vi "2-Position Single Solenoid Control.vi"(6 "Sensor Analog Status":sgl format="%#_13g", 7 "Sensor Digital Status":bool, 9 "Feedback":T5(ring), 10 "Action":T4(ring), 11 "PneumaticsDevRefIn":T1={"Pneumatic State Reference"=refnum, "SolenoidDevRef"={"DevStatus"={"status"=FALSE, "code"=0, "source"=""}, "Pneumatics Control Module"=0, "Forward Solenoid Channel"=enum."Invalid", "Reverse Solenoid Channel"=enum."Invalid"}, "Pneumatic Configuration reference"=refnum}) -> (1 "Action Complete":bool, 2 "Solenoid Position":bool, 3 "PneumaticsDevRefOut":T1={"Pneumatic State Reference"=refnum, "SolenoidDevRef"={"DevStatus"={"status"=FALSE, "code"=0, "source"=""}, "Pneumatics Control Module"=0, "Forward Solenoid Channel"=enum."Invalid", "Reverse Solenoid Channel"=enum."Invalid"}, "Pneumatic Configuration reference"=refnum})   [LabVIEW 2014]
uses:
  <userlib>/836 Library/Pneumatics/Pneumatics/836_PneumaticsDevRef.ctl
  <userlib>/836 Library/Pneumatics/Pneumatics/Pneumatic State.ctl
  <userlib>/836 Library/Pneumatics/Pneumatics/StateMachine.ctl
  <vilib>/Rock Robotics/WPI/Solenoid/WPI_SolenoidDevRef.ctl
  <vilib>/Rock Robotics/WPI/Solenoid/WPI_SolenoidChannel.ctl
  <userlib>/836 Library/Pneumatics/Pneumatics/Pneumatic Configuration.ctl
  <vilib>/Rock Robotics/WPI/Solenoid/WPI_SolenoidValue.ctl
  <vilib>/Rock Robotics/WPI/Solenoid/WPI_SolenoidSetEnum.vi
panel:
  out "error IO":errorcluster
  out "Error Out":errorcluster
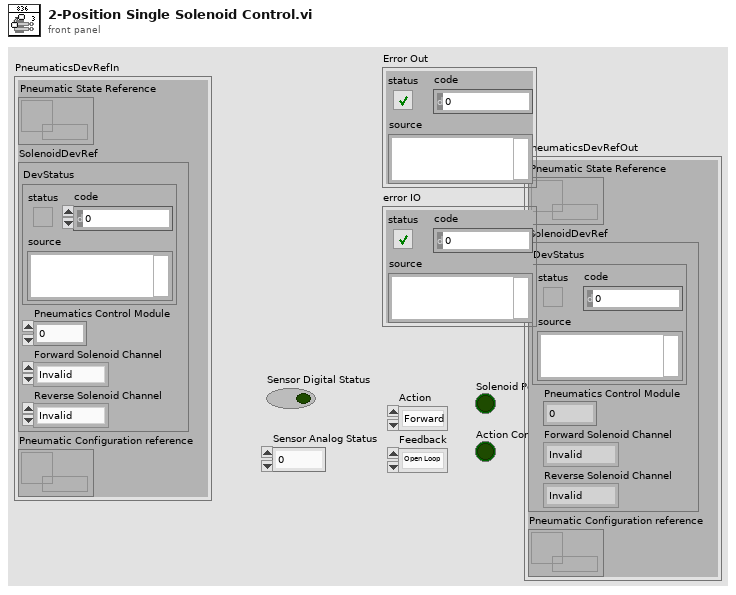
[diagram p1: front panel]
types:
  T1 = typedef "836_PneumaticsDevRef.ctl" = cluster{"Pneumatic State Reference":refnum<data-value>, "SolenoidDevRef":T2, "Pneumatic Configuration reference":refnum<data-value>}
  T2 = typedef "WPI_SolenoidDevRef.ctl" = cluster{"DevStatus":errorcluster, "Pneumatics Control Module":u8, "Forward Solenoid Channel":T3, "Reverse Solenoid Channel":T3}
  T3 = typedef "WPI_SolenoidChannel.ctl" = enum8{"Solenoid 0", "Solenoid 1", "Solenoid 2", "Solenoid 3", "Solenoid 4", "Solenoid 5", "Solenoid 6", "Solenoid 7", "Invalid"}
  T4 = enum16{"Forward", "Back", "Toggle", "Status", "Float"}
  T5 = enum16{"Open Loop", "Analog", "Digital", "Timed"}
  T6 = typedef "WPI_SolenoidValue.ctl" = enum16{"Off", "On", "Forward", "Reverse"}
  T7 = typedef "StateMachine.ctl" = enum8{"Status", "Forward", "Back", "Toggle", "Timed Forward", "Timed Back", "Analog Forwad", "Analog Back", "Digital Forward", "Digital Back", "Off", "Float"}
  T8 = typedef "Pneumatic State.ctl" = cluster{"Position":bool, "Initialize":bool, "Current State":T7, "Multiuse Timer":u32}
  T9 = typedef "Pneumatic Configuration.ctl" = cluster{"Time Forward":u32, "Time Back":u32, "Digital Forward Samples":u32, "Digital Backward Samples":u32, "Analog Forward Settling Time":u32, "Analog Backward Settling Time":u32, "Analog Forward Threshold":sgl, "Analog Backward Threshold":sgl}
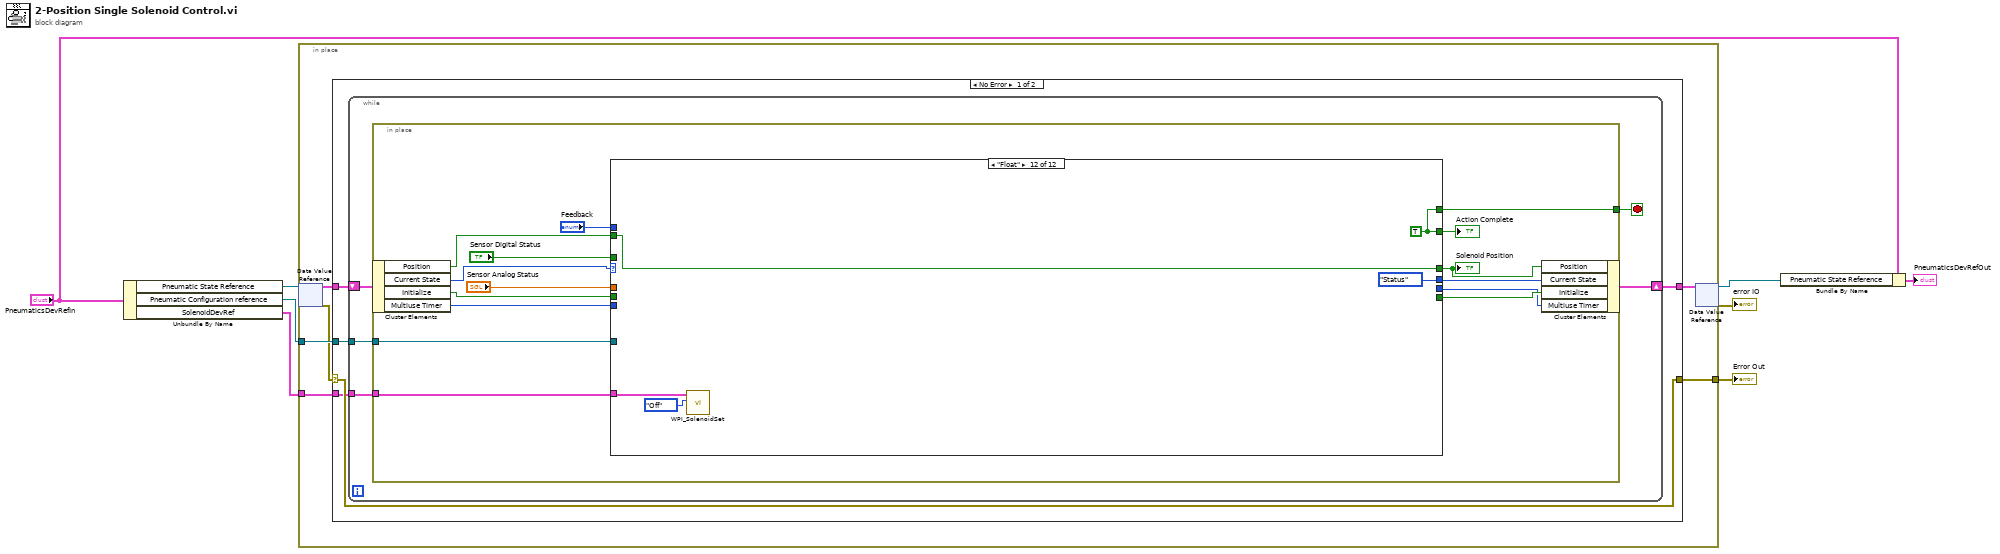
[diagram p0: block diagram]
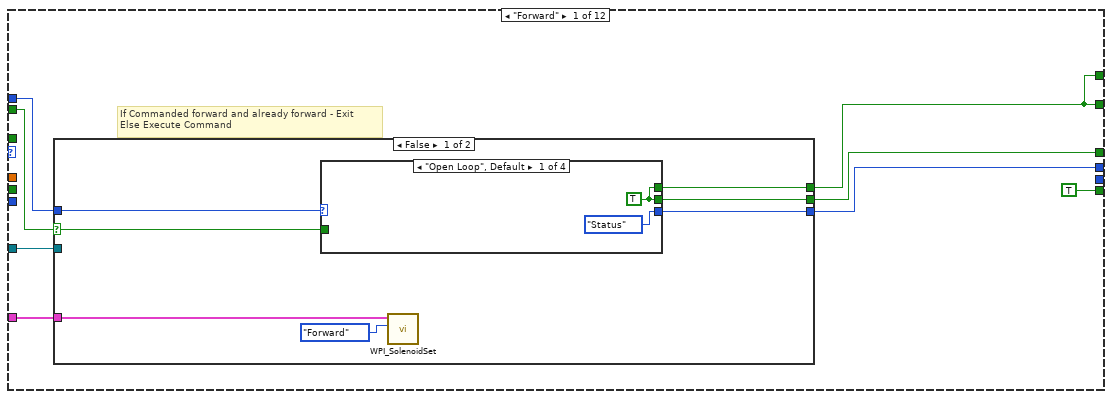
[diagram p2: hidden frame]
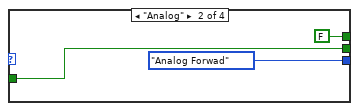
[diagram p3: hidden frame]
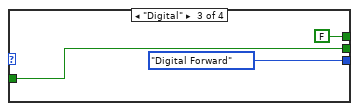
[diagram p4: hidden frame]
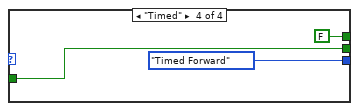
[diagram p5: hidden frame]
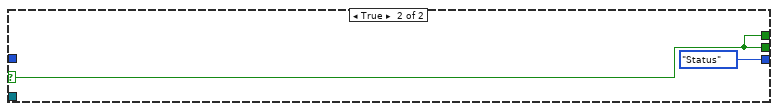
[diagram p6: hidden frame]
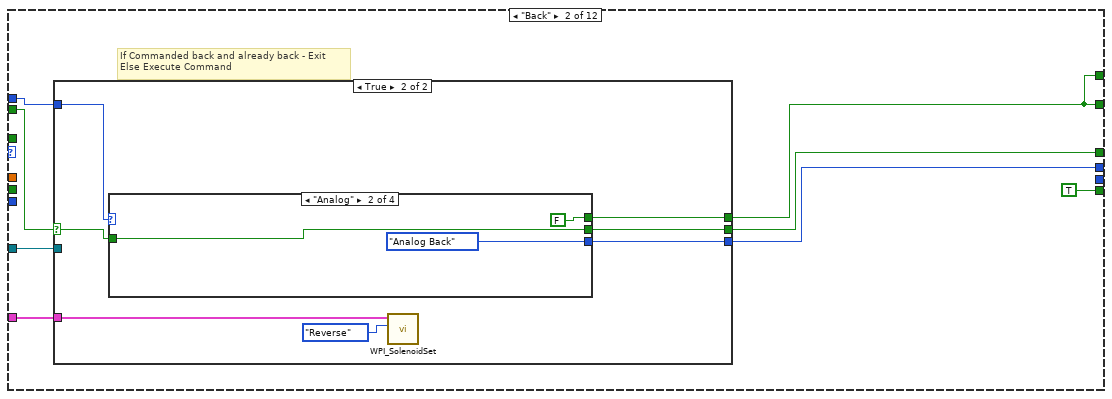
[diagram p7: hidden frame]
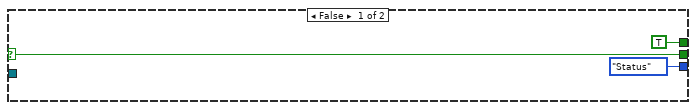
[diagram p8: hidden frame]
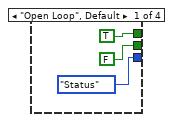
[diagram p9: hidden frame]
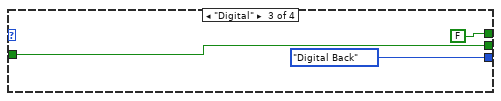
[diagram p10: hidden frame]
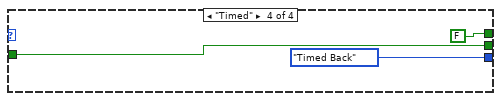
[diagram p11: hidden frame]
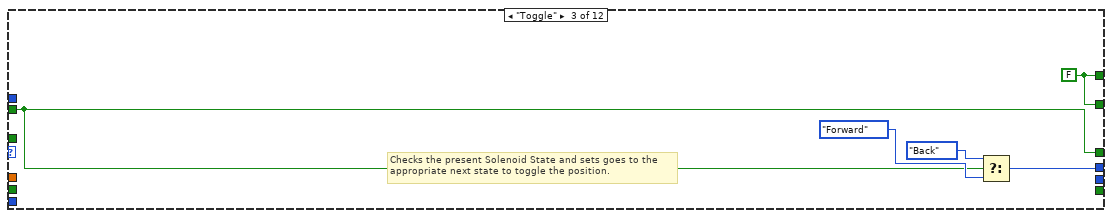
[diagram p12: hidden frame]
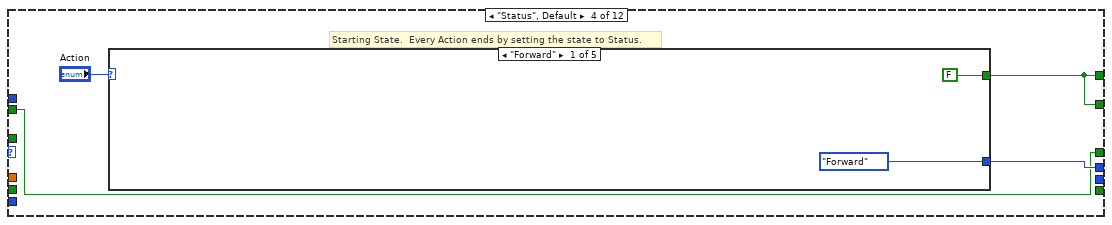
[diagram p13: hidden frame]
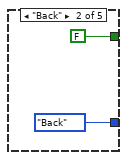
[diagram p14: hidden frame]
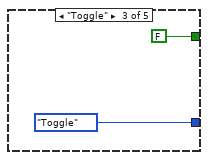
[diagram p15: hidden frame]
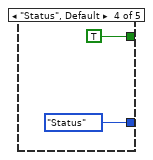
[diagram p16: hidden frame]
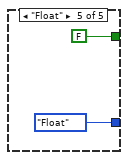
[diagram p17: hidden frame]
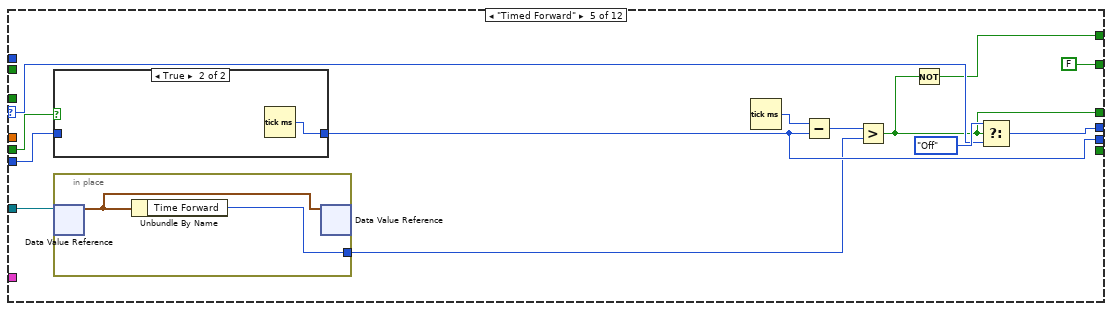
[diagram p18: hidden frame]
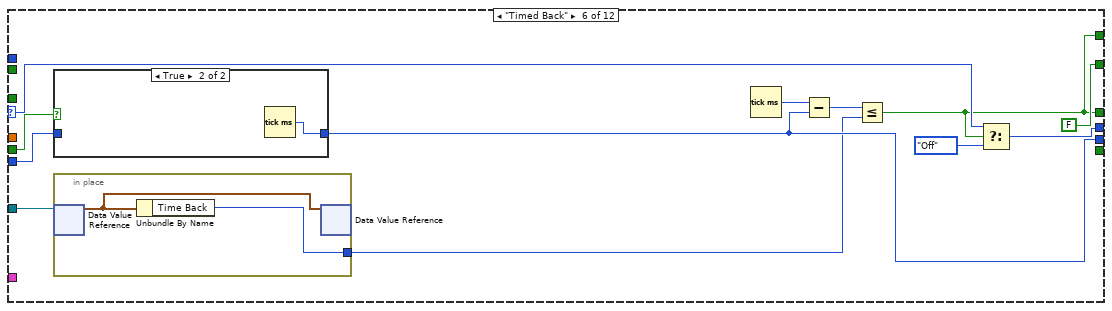
[diagram p20: hidden frame]
diagram:
  n1 = Unbundle By Name("PneumaticsDevRefIn") -> ("Pneumatic State Reference"=w8:refnum<data-value>, "Pneumatic Configuration reference"=w7:refnum<data-value>, "SolenoidDevRef"=w1:T2)
  n2 = in-place {
    in-place-border: w7 -> [w13]
    in-place-border: [w10] -> w3
    in-place-border: w1 -> [w9]
    n3 = in-place-dvr #1(w8) -> (w14:T8, w11:errorcluster)
    n4 = case shown="No Error" w11 {
      selector: w11 -> [w17 w238]
      tunnel: w14 -> [w19 w239]
      tunnel: w13 -> [w18 _]
      tunnel: [w16 w239] -> w12
      tunnel: [w17 w238] -> w10
      tunnel: w9 -> [w15 _]
      frame No Error {
        n5 = while {
          tunnel: w18 -> [w23]
          shift-right: [w21] -> w16
          shift-left: w19 -> [w24]
          tunnel: w15 -> [w20]
          stop <- w22 stop-if-true
          n6 = in-place {
            in-place-border: w23 -> [w31]
            in-place-border: [w27] -> w22
            in-place-border: w20 -> [w25]
            n7 = in-place-cluster #2(w24) -> ("Position"=w35:bool, "Current State"=w29:T7, "Initialize"=w34:bool, "Multiuse Timer"=w30:u32)
            n8 = case shown="\"Float\"" w29 {
              selector: w29 -> [_ _ _ _ w127 w142 w159 w184 w204 w218 _ _]
              tunnel: [w45 w73 w98 w104 w119 w136 w154 w175 w195 w213 w228 w235] -> w27
              tunnel: "Feedback" -> [w47 w75 _ _ _ _ _ _ _ _ _ _]
              tunnel: w35 -> [w43 w72 w101 w105 _ _ _ _ _ _ w229 w236]
              tunnel: [w46 w74 w101 w105 w120 w136 w153 w175 w196 w213 w229 w236] -> w33
              tunnel: "Sensor Digital Status" -> [_ _ _ _ _ _ _ _ w206 w221 _ _]
              tunnel: [w44 w71 w99 w106 w128 w145 w166 w187 w207 w222 StateMachine."Status" StateMachine."Status"] -> w32
              tunnel: "Sensor Analog Status" -> [_ _ _ _ _ _ w163 w181 _ _ _ _]
              tunnel: w34 -> [_ _ _ _ w121 w137 w155 w176 w198 w214 _ _]
              tunnel: [w45 w73 w98 w104 FALSE FALSE FALSE FALSE FALSE FALSE w228 w235] -> w36
              tunnel: w30 -> [_ _ _ _ w122 w138 w156 w177 w199 w215 _ _]
              tunnel: [_ _ _ _ w123 w139 w157 w178 w200 w216 _ _] -> w26
              tunnel: w31 -> [w42 w70 _ _ w118 w135 w152 w174 w194 w212 _ _]
              tunnel: [TRUE TRUE _ _ _ _ _ _ _ _ _ _] -> w28
              tunnel: w25 -> [w40 w68 _ _ _ _ _ _ _ _ w227 w234]
              frame "Forward" {
                # "If Commanded forward and already forward - Exit\nElse Execute Command"
                n9 = case shown="False" w43 {
                  selector: w43 -> [w50 w66]
                  tunnel: w47 -> [w54 _]
                  tunnel: [w53 w66] -> w46
                  tunnel: [w52 w66] -> w45
                  tunnel: [w51 StateMachine."Status"] -> w44
                  tunnel: w42 -> [_ _]
                  tunnel: w40 -> [w48 _]
                  frame False {
                    n10 = case shown="\"Open Loop\", Default" w54 {
                      tunnel: [w55 FALSE FALSE FALSE] -> w52
                      tunnel: [StateMachine."Status" StateMachine."Analog Forwad" StateMachine."Digital Forward" StateMachine."Timed Forward"] -> w51
                      tunnel: w50 -> [_ w57 w60 w63]
                      tunnel: [w55 w57 w60 w63] -> w53
                      frame "Open Loop", Default {
                        w55 = TRUE
                      }
                      frame "Analog" {
                      }
                      frame "Digital" {
                      }
                      frame "Timed" {
                      }
                    }
                    n11 = call-poly <vilib>:"WPI_SolenoidSet.vi"("Value"=WPI_SolenoidValue."Forward" ("Value 3"), "SolenoidDevRef"=w48) -> ()  [unwired: 8 in, 2 out]
                  }
                  frame True {
                  }
                }
              }
              frame "Back" {
                # "If Commanded back and already back - Exit\nElse Execute Command"
                n12 = case shown="True" w72 {
                  selector: w72 -> [w76 w81]
                  tunnel: w75 -> [_ w85]
                  tunnel: [w76 w84] -> w74
                  tunnel: [TRUE w83] -> w73
                  tunnel: [StateMachine."Status" w82] -> w71
                  tunnel: w70 -> [_ _]
                  tunnel: w68 -> [_ w79]
                  frame False {
                  }
                  frame True {
                    n13 = case shown="\"Analog\"" w85 {
                      tunnel: [TRUE FALSE FALSE FALSE] -> w83
                      tunnel: [StateMachine."Status" StateMachine."Analog Back" StateMachine."Digital Back" StateMachine."Timed Back"] -> w82
                      tunnel: [FALSE w89 w92 w95] -> w84
                      tunnel: w81 -> [_ w89 w92 w95]
                      frame "Open Loop", Default {
                      }
                      frame "Analog" {
                      }
                      frame "Digital" {
                      }
                      frame "Timed" {
                      }
                    }
                    n14 = call-poly <vilib>:"WPI_SolenoidSet.vi"("Value"=WPI_SolenoidValue."Reverse" ("Value 3"), "SolenoidDevRef"=w79) -> ()  [unwired: 8 in, 2 out]
                  }
                }
              }
              frame "Toggle" {
                w98 = FALSE
                # "Checks the present Solenoid State and sets goes to the\nappropriate next state to toggle the position."
                n15 = Select(t=StateMachine."Back", s=w101, f=StateMachine."Forward") -> (s? t:f=w99:T7)
              }
              frame "Status", Default {
                # "Starting State.  Every Action ends by setting the state to Status."
                n16 = case shown="\"Forward\"" "Action" {
                  tunnel: [FALSE FALSE FALSE TRUE FALSE] -> w104
                  tunnel: [StateMachine."Forward" StateMachine."Back" StateMachine."Toggle" StateMachine."Status" StateMachine."Float"] -> w106
                  frame "Forward" {
                  }
                  frame "Back" {
                  }
                  frame "Toggle" {
                  }
                  frame "Status", Default {
                  }
                  frame "Float" {
                  }
                }
              }
              frame "Timed Forward" {
                n17 = case shown="True" w121 {
                  tunnel: [w132 w133] -> w123
                  tunnel: w122 -> [w132 _]
                  frame False {
                  }
                  frame True {
                    n18 = Tick Count (ms)() -> (millisecond timer value=w133:u32)
                  }
                }
                n19 = in-place {
                  in-place-border: [w130] -> w117
                  n20 = in-place-dvr #3(w118) -> (w131:T9)  [unwired: 1 out]
                  n21 = Unbundle By Name(w131) -> ("Time Forward"=w130:u32)
                  n22 = in-place-dvr #3(w131) -> ()  [unwired: 2 out]
                }
                n23 = Tick Count (ms)() -> (millisecond timer value=w125:u32)
                n24 = Subtract(x=w125, y=w123) -> (x-y=w126:u32)
                n25 = Greater?(x=w126, y=w117) -> (0:w120:bool)
                n26 = Not(x=w120) -> (.not. x?=w119:bool)
                n27 = Select(t=StateMachine."Off", s=w120, f=w127) -> (s? t:f=w128:T7)
              }
              frame "Timed Back" {
                n28 = case shown="True" w137 {
                  tunnel: [w148 w149] -> w139
                  tunnel: w138 -> [w148 _]
                  frame False {
                  }
                  frame True {
                    n29 = Tick Count (ms)() -> (millisecond timer value=w149:u32)
                  }
                }
                n30 = in-place {
                  in-place-border: [w146] -> w134
                  n31 = in-place-dvr #4(w135) -> (w147:T9)  [unwired: 1 out]
                  n32 = Unbundle By Name(w147) -> ("Time Back"=w146:u32)
                  n33 = in-place-dvr #4(w147) -> ()  [unwired: 2 out]
                }
                n34 = Tick Count (ms)() -> (millisecond timer value=w141:u32)
                n35 = Subtract(x=w141, y=w139) -> (x-y=w144:u32)
                n36 = Less Or Equal?(x=w144, y=w134) -> (x <= y?=w136:bool)
                n37 = Select(t=w142, s=w136, f=StateMachine."Off") -> (s? t:f=w145:T7)
              }
              frame "Analog Forwad" {
                n38 = in-place {
                  in-place-border: [w168] -> w151
                  in-place-border: [w167] -> w150
                  n39 = in-place-dvr #5(w152) -> (w169:T9)  [unwired: 1 out]
                  n40 = Unbundle By Name(w169) -> ("Analog Forward Settling Time"=w168:u32, "Analog Forward Threshold"=w167:sgl)
                  n41 = in-place-dvr #5(w169) -> ()  [unwired: 2 out]
                }
                n42 = Greater?(x=w150, y=w163) -> (0:w162:bool)
                n43 = Or(x=w162, y=w155) -> (x .or. y?=w164:bool)
                n44 = case shown="True" w164 {
                  tunnel: [w170 w171] -> w157
                  tunnel: w156 -> [w170 _]
                  frame False {
                  }
                  frame True {
                    n45 = Tick Count (ms)() -> (millisecond timer value=w171:u32)
                  }
                }
                n46 = Tick Count (ms)() -> (millisecond timer value=w165:u32)
                n47 = Subtract(x=w165, y=w157) -> (x-y=w161:u32)
                n48 = Greater?(x=w161, y=w151) -> (0:w153:bool)
                n49 = Not(x=w153) -> (.not. x?=w154:bool)
                n50 = Select(t=StateMachine."Off", s=w153, f=w159) -> (s? t:f=w166:T7)
              }
              frame "Analog Back" {
                n51 = in-place {
                  in-place-border: [w189] -> w173
                  in-place-border: [w188] -> w172
                  n52 = in-place-dvr #6(w174) -> (w190:T9)  [unwired: 1 out]
                  n53 = Unbundle By Name(w190) -> ("Analog Backward Threshold"=w189:sgl, "Analog Backward Settling Time"=w188:u32)
                  n54 = in-place-dvr #6(w190) -> ()  [unwired: 2 out]
                }
                n55 = Greater Or Equal?(x=w181, y=w173) -> (x >= y?=w180:bool)
                n56 = Or(x=w176, y=w180) -> (x .or. y?=w182:bool)
                n57 = case shown="True" w182 {
                  tunnel: [w191 w192] -> w178
                  tunnel: w177 -> [w191 _]
                  frame False {
                  }
                  frame True {
                    n58 = Tick Count (ms)() -> (millisecond timer value=w192:u32)
                  }
                }
                n59 = Tick Count (ms)() -> (millisecond timer value=w183:u32)
                n60 = Subtract(x=w183, y=w178) -> (x-y=w186:u32)
                n61 = Less?(x=w186, y=w172) -> (x < y?=w175:bool)
                n62 = Select(t=w184, s=w175, f=StateMachine."Off") -> (s? t:f=w187:T7)
              }
              frame "Digital Forward" {
                n63 = in-place {
                  in-place-border: [w209] -> w193
                  n64 = in-place-dvr #7(w194) -> (w210:T9)  [unwired: 1 out]
                  n65 = Unbundle By Name(w210) -> ("Digital Forward Samples"=w209:u32)
                  n66 = in-place-dvr #7(w210) -> ()  [unwired: 2 out]
                }
                n67 = Not(x=w198) -> (.not. x?=w197:bool)
                n68 = And(x=w206, y=w197) -> (x .and. y?=w205:bool)
                n69 = Increment(x=w199) -> (x+1=w202:u32)
                n70 = Select(t=w202, s=w205, f=u32 0 ("t")) -> (s? t:f=w200:u32)
                n71 = Greater Or Equal?(x=w200, y=w193) -> (x >= y?=w196:bool)
                n72 = Not(x=w196) -> (.not. x?=w195:bool)
                n73 = Select(t=StateMachine."Off", s=w196, f=w204) -> (s? t:f=w207:T7)
              }
              frame "Digital Back" {
                n74 = in-place {
                  in-place-border: [w225] -> w211
                  n75 = in-place-dvr #8(w212) -> (w226:T9)  [unwired: 1 out]
                  n76 = Unbundle By Name(w226) -> ("Digital Backward Samples"=w225:u32)
                  n77 = in-place-dvr #8(w226) -> ()  [unwired: 2 out]
                }
                n78 = Not Or(1:w221, 2:w214) -> (0:w223:bool)
                n79 = Increment(x=w215) -> (x+1=w220:u32)
                n80 = Select(t=w220, s=w223, f=u32 0 ("t")) -> (s? t:f=w216:u32)
                n81 = Less?(x=w216, y=w211) -> (x < y?=w213:bool)
                n82 = Select(t=w218, s=w213, f=StateMachine."Off") -> (s? t:f=w222:T7)
              }
              frame "Off" {
                w228 = TRUE
                # "Disabled so this VI can be used for 3-Position Solenoids"
                n83 = disable-structure shown="Disabled" {
                  disable-tunnel: w227 -> [w231 _]
                  frame Disabled {
                    n84 = call-poly <vilib>:"WPI_SolenoidSet.vi"("Value"=WPI_SolenoidValue."Off" ("Value 3"), "SolenoidDevRef"=w231) -> ()  [unwired: 8 in, 2 out]
                  }
                  frame Enabled {
                  }
                }
              }
              frame "Float" {
                w235 = TRUE
                n85 = call-poly <vilib>:"WPI_SolenoidSet.vi"("Value"=WPI_SolenoidValue."Off" ("Value 3"), "SolenoidDevRef"=w234) -> ()  [unwired: 8 in, 2 out]
              }
            }
            "Solenoid Position" <- w33
            "Action Complete" <- w36
            n86 = in-place-cluster #2("Position"=w33, "Current State"=w32, "Initialize"=w28, "Multiuse Timer"=w26) -> (w21:T8)
          }
        }
      }
      frame Error {
      }
    }
    n87 = in-place-dvr #1(w12) -> (w4:refnum<data-value>, →"error IO":errorcluster)
  }
  "Error Out" <- w3
  n88 = Bundle By Name(cluster="PneumaticsDevRefIn", "Pneumatic State Reference"=w4) -> (→"PneumaticsDevRefOut":T1)
